vi "USBImageContinuousV1.3.vi"() -> ()   [LabVIEW 2017]
uses:
  C:/Program Files (x86)/National Instruments/LabVIEW 2019/ATMCD32D.dll
  <vilib>/Utility/file.llb/Write Delimited Spreadsheet (I64).vi
panel:
  in  "Tab Control":T1(tab)
  out "Expected position on spectrometer (pixels):":dbl
  in  "Harmonic":dbl min=10.0 max=40.0
  out "l (nm)":dbl
  out "E (J)":dbl
  out "E (eV)":dbl
  out "Nearest Harmonic of 800nm":dbl
  out "Cursor Position (pixels)":dbl
  out "Distance to nearest harmonic of 800nm (pixels)":dbl
  in  "Grating:":u16(ring) items=["Shimadzu 30-006  "]
  in  "Laser:":u16(ring) items=["800nm  "]
  in  "Trigger":u32(ring) items=["Internal", "External"]
  out "Initialize":u32
  in  "Exposure Time (secs)":sgl format="%.2f"
  out "Calculated Exposure Value":sgl format="%.5f"
  out "Get Acquired Data":u32
  out "Start Acquisition":u32
  out "Detector X Pixels":i32
  out "Check Timings":u32
  out "Set Acquisition Mode":u32
  out "Set Readout Mode":u32
  out "Set Trigger Mode":u32
  out "Set Exposure Time":u32
  out "Get Detector":u32
  out "Detector Y Pixels":i32
  out "Shut Down":u32
  out "Set Gate Mode":u32
  out "Set Image":u32
  out "Raw Image From Camera":i32[][](graph)
  out "Vertical Binned Waveform Graph":i32[](graph)
  out "Get Status":u32
  in  "Stop":bool
  in  "?":bool
  out "Camera Status:":bool
  out "Last Image Saved:":string
  in  "Caibration Date":u16(ring) items=["first calibration - 7/31", "7/31-current"]
  out "Caibration Date: indicator:":u16(ring) items=["first calibration - 7/31", "7/31-current"]
  out "Wavelength Graph (nm)":cluster{"No prefix":dbl, i32}[](graph)
  out "Energy Graph (eV)":cluster{"eV":dbl, i32}[](graph)
  out "Harmonics Graph":cluster{"No prefix":dbl, i32}[](graph)
  out "Status":u32
  # "Status"
  # "Return values"
  # "Acquisition Mode: Single Scan\nReadout Mode: Full Resolution Image"
  # "XUV Spectrometer Control VI"
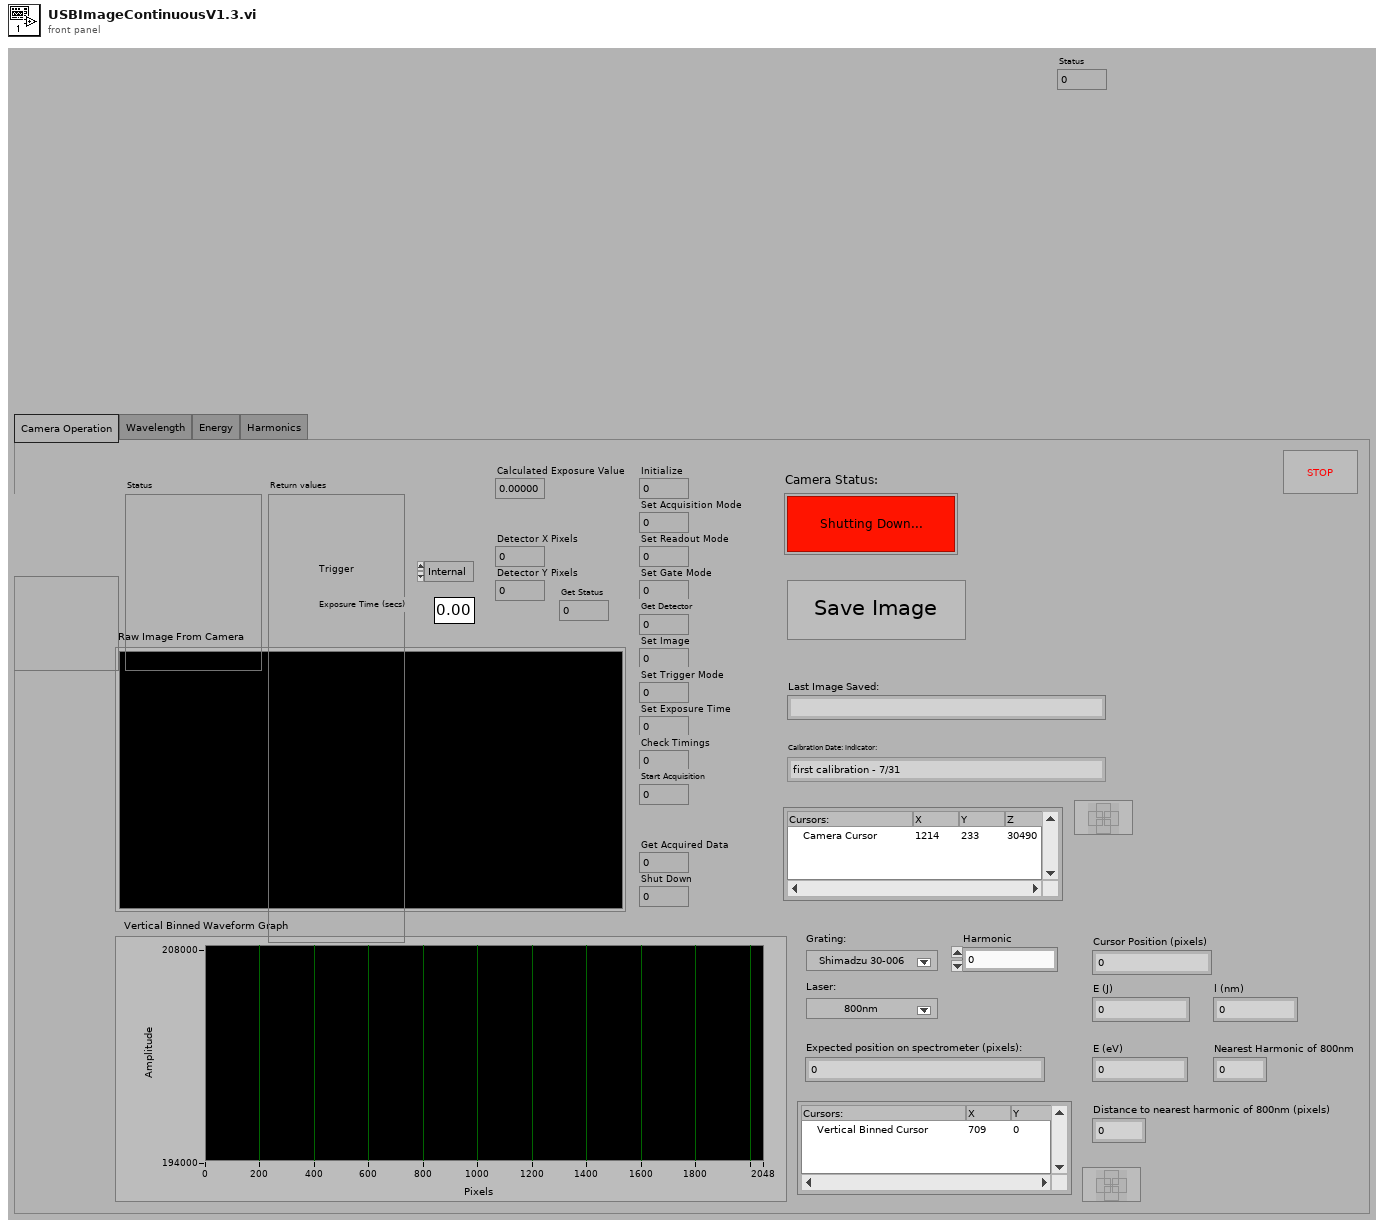
[diagram p1: front panel]
types:
  T1 = enum32{"Camera Operation", "Wavelength", "Energy", "Harmonics"}
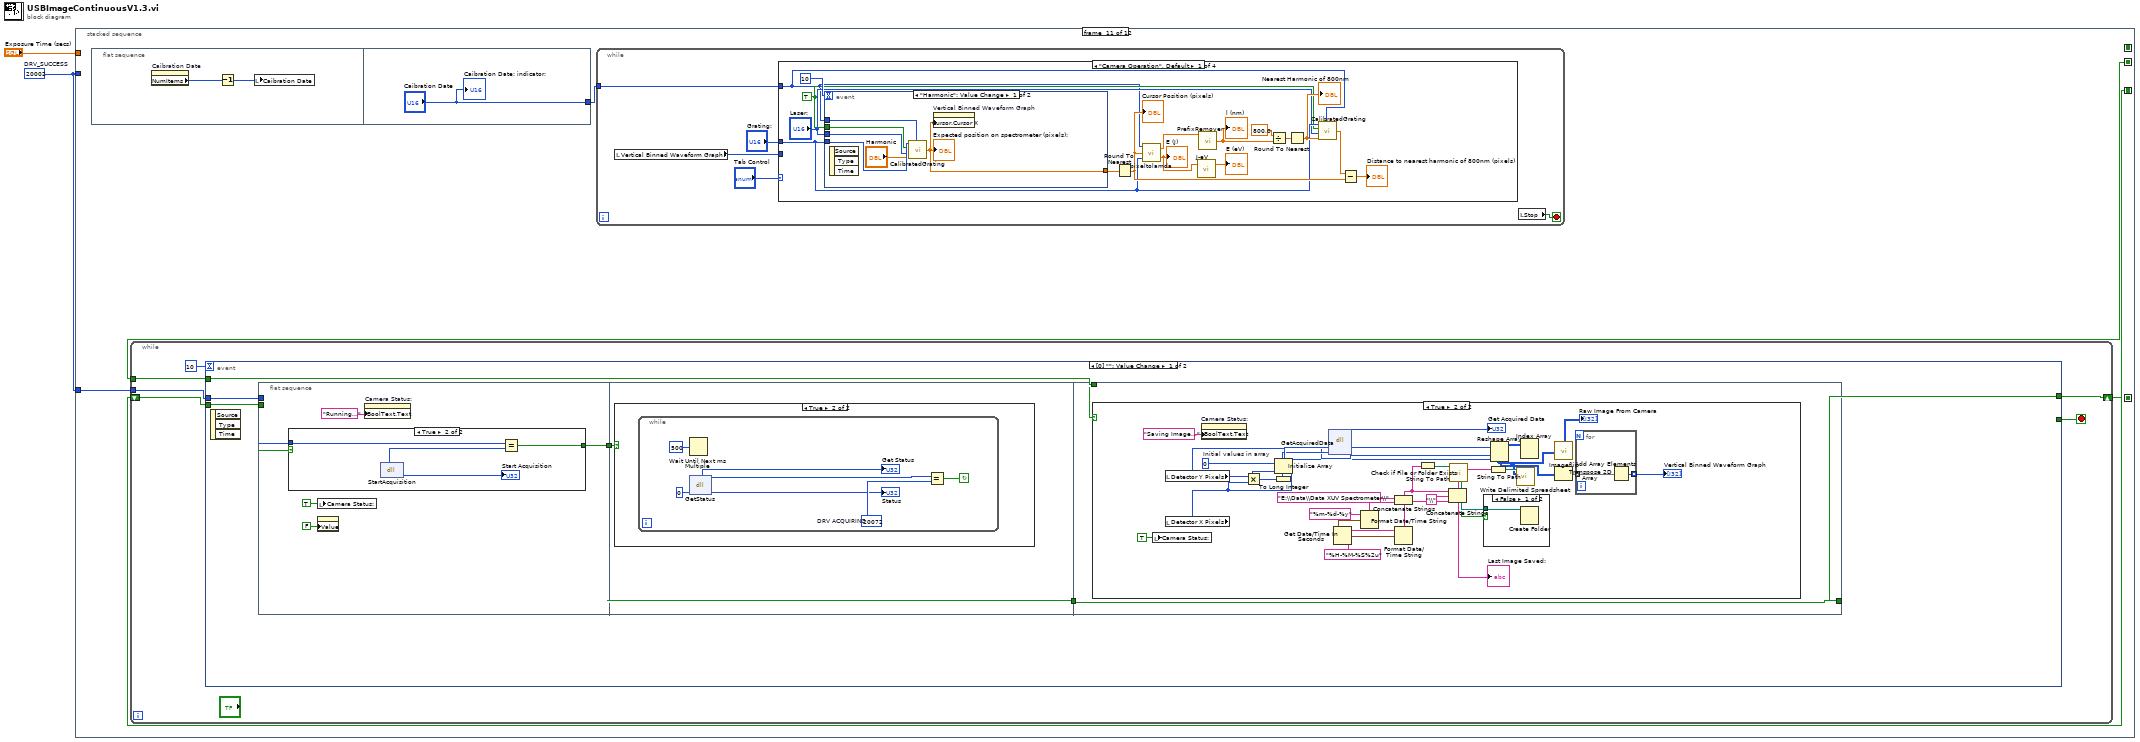
[diagram p0: block diagram]
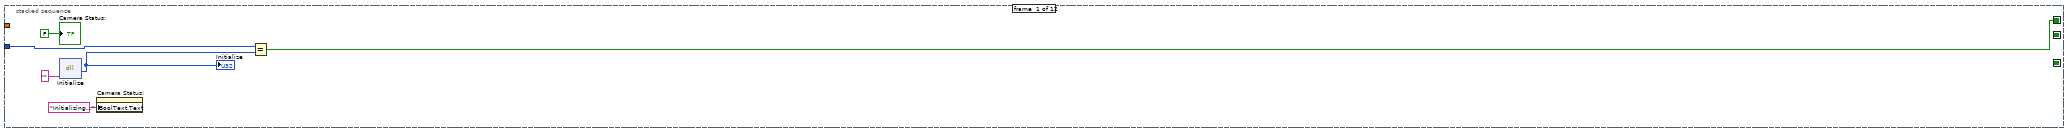
[diagram p2: hidden frame]
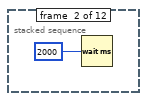
[diagram p3: hidden frame]
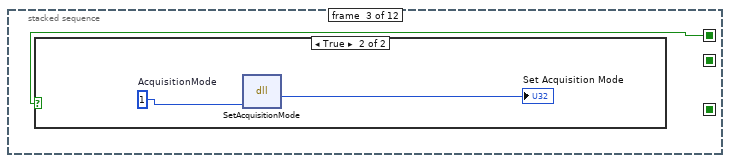
[diagram p4: hidden frame]
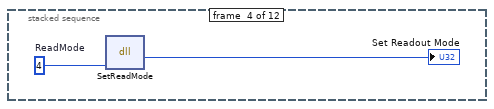
[diagram p6: hidden frame]
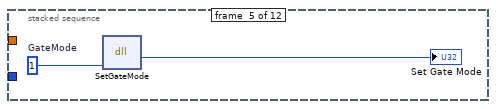
[diagram p7: hidden frame]
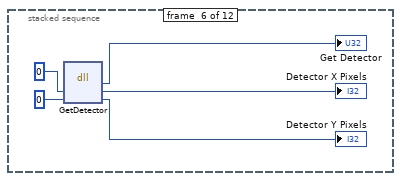
[diagram p8: hidden frame]
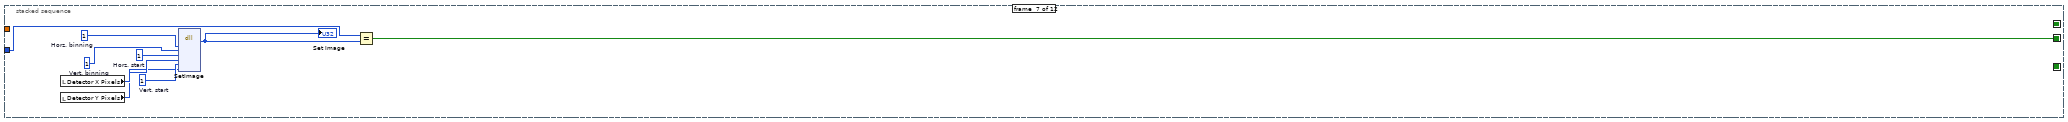
[diagram p9: hidden frame]
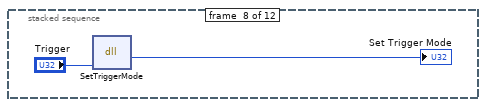
[diagram p10: hidden frame]
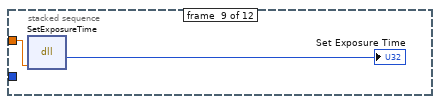
[diagram p11: hidden frame]
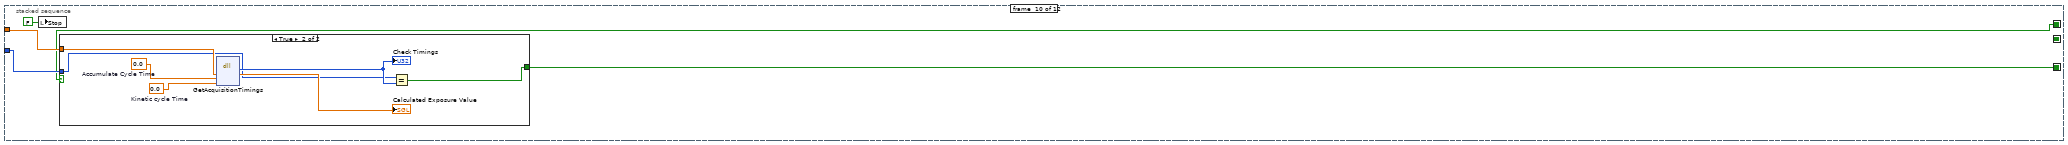
[diagram p12: hidden frame]
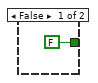
[diagram p13: hidden frame]
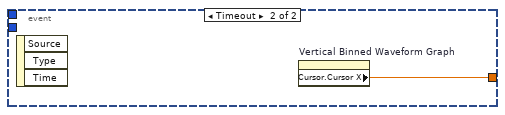
[diagram p14: hidden frame]
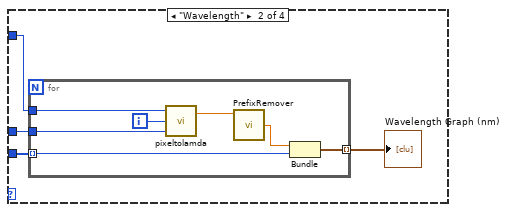
[diagram p15: hidden frame]
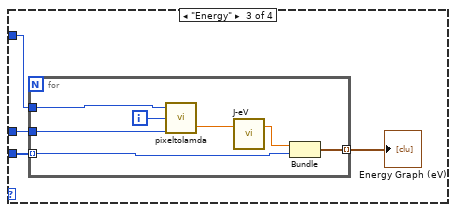
[diagram p16: hidden frame]
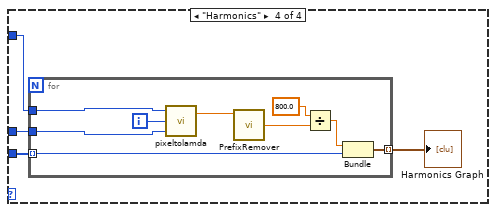
[diagram p17: hidden frame]
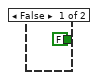
[diagram p18: hidden frame]
diagram:
  w1 = 20002  # DRV_SUCCESS
  n1 = stacked-sequence {
    seq-local: [w6 _ _ _ _ _ _ _ _ _ _ _] -> [_ _ w10 _ _ _ _ _ _ w36 _ w233]
    seq-local: [_ _ _ _ _ _ _ _ _ w37 _ _] -> [_ _ _ _ _ _ _ _ _ _ w52 _]
    seq-local: [_ _ _ _ _ _ _ _ _ _ w50 _] -> [_ _ _ _ _ _ _ _ _ _ _ _]
    seq-local: [_ _ _ _ _ _ w22 _ _ _ _ _] -> [_ _ _ _ _ _ _ _ _ _ w49 _]
    tunnel: "Exposure Time (secs)" -> [_ _ _ _ _ _ _ _ w34 w39 _ _]
    tunnel: w1 -> [w7 _ _ _ _ _ w24 _ _ w38 _ _]
    tunnel: w1 -> [_ _ _ _ _ _ _ _ _ _ w51 _]
    frame #0 {
      n2 = dll-call lib="C:/Program Files (x86)/National Instruments/LabVIEW 2019/atmcd32d.dll" fn="Initialize" label="Call Library Function Initialize"("") -> (w8:u32)  [unwired: 4 in, 2 out]
      "Initialize" <- w8
      n3 = property on="Camera Status:" class="Bool (strict)"("BoolText.Text"="Initializing..." ("String")) -> ()  [unwired: 2 in, 2 out]
      n4 = Equal?(x=w7, y=w8) -> (x = y?=w6:bool)
      "Camera Status:" <- FALSE ("Camera Status:")
    }
    frame #1 {
      n5 = Wait (ms)(milliseconds to wait=u32 2000) -> ()  [unwired: 1 out]
    }
    frame #2 {
      n6 = case shown="True" w10 {
        frame False {
        }
        frame True {
          w12 = u16 1  # AcquisitionMode
          n7 = dll-call lib="C:/Program Files (x86)/National Instruments/LabVIEW 2019/atmcd32d.dll" fn="SetAcquisitionMode" label="Call Library Function SetAcquisitionMode"(w12) -> (→"Set Acquisition Mode":u32)  [unwired: 4 in, 2 out]
        }
      }
    }
    frame #3 {
      w14 = u16 4  # ReadMode
      n8 = dll-call lib="C:/Program Files (x86)/National Instruments/LabVIEW 2019/atmcd32d.dll" fn="SetReadMode" label="Call Library Function SetReadMode"(w14) -> (→"Set Readout Mode":u32)  [unwired: 4 in, 2 out]
    }
    frame #4 {
      w16 = u16 1  # GateMode
      n9 = dll-call lib="C:/Program Files (x86)/National Instruments/LabVIEW 2019/atmcd32d.dll" fn="SetGateMode" label="Call Library Function SetGateMode"(w16) -> (→"Set Gate Mode":u32)  [unwired: 4 in, 2 out]
    }
    frame #5 {
      n10 = dll-call lib="C:/Program Files (x86)/National Instruments/LabVIEW 2019/atmcd32d.dll" fn="GetDetector" label="Call Library FunctionGetDetector"(i16 0, i16 0) -> (→"Get Detector":u32, →"Detector X Pixels":i32, →"Detector Y Pixels":i32)  [unwired: 3 in, 2 out]
    }
    frame #6 {
      w27 = u16 1  # Vert. start
      w28 = u16 1  # Horz. start
      w29 = u16 1  # Vert. binning
      w30 = u16 1  # Horz. binning
      n11 = local read "Detector X Pixels"() -> (w26:i32)
      n12 = local read "Detector Y Pixels"() -> (w25:i32)
      n13 = dll-call lib="C:/Program Files (x86)/National Instruments/LabVIEW 2019/atmcd32d.dll" fn="SetImage" label="Call Library Function SetImage"(w30, w29, w28, w26, w27, w25) -> (w23:u32)  [unwired: 9 in, 2 out]
      "Set Image" <- w23
      n14 = Equal?(x=w24, y=w23) -> (x = y?=w22:bool)
    }
    frame #7 {
      n15 = dll-call lib="C:/Program Files (x86)/National Instruments/LabVIEW 2019/atmcd32d.dll" fn="SetTriggerMode" label="Call Library Function SetTrigger Mode"("Trigger") -> (→"Set Trigger Mode":u32)  [unwired: 4 in, 2 out]
    }
    frame #8 {
      n16 = dll-call lib="C:/Program Files (x86)/National Instruments/LabVIEW 2019/atmcd32d.dll" fn="SetExposureTime" label="Call Library FunctionSet Exposure Time"(w34) -> (→"Set Exposure Time":u32)  [unwired: 4 in, 2 out]
    }
    frame #9 {
      n17 = local write "Stop"(FALSE ("Stop")) -> ()
      n18 = case shown="True" w36 {
        tunnel: w39 -> [_ w44]
        tunnel: w38 -> [_ w41]
        tunnel: [FALSE w43] -> w37
        frame False {
        }
        frame True {
          w46 = sgl 0.0  # Accumulate Cycle Time
          w47 = sgl 0.0  # Kinetic cycle Time
          n19 = dll-call lib="C:/Program Files (x86)/National Instruments/LabVIEW 2019/atmcd32d.dll" fn="GetAcquisitionTimings" label="Call Library Function Check Timings"(w44, w46, w47) -> (w42:u32, →"Calculated Exposure Value":sgl)  [unwired: 5 in, 2 out]
          "Check Timings" <- w42
          n20 = Equal?(x=w41, y=w42) -> (x = y?=w43:bool)
        }
      }
    }
    frame #10 {
      n21 = flat-sequence {
        tunnel: ["Caibration Date"] -> w48
        frame #0 {
          n22 = property on="Caibration Date" class="Ring (strict)"() -> ("NumItems"=w54:u32)  [unwired: 2 in, 2 out]
          n23 = Decrement(x=w54) -> (x-1=w53:u32)
          n24 = local write "Caibration Date"(w53) -> ()
        }
        frame #1 {
          "Caibration Date: indicator:" <- "Caibration Date"
        }
      }
      n25 = while {
        tunnel: w51 -> [w123]
        tunnel: w49 -> [w121]
        shift-right: [w122] -> w50
        shift-left: w52 -> [w124]
        stop <- w119 stop-if-true
        n26 = event shown="[0] \"\": Value Change" {
          selector: _ -> [_ _]
          dyn-events: _ -> [_ _]
          timeout: 10 -> [_ _]
          tunnel: w124 -> [w128 w185]
          tunnel: w123 -> [w127 w184]
          tunnel: [w126 w183] -> w122
          tunnel: w121 -> [w125 w182]
          tunnel: [_ w181] -> w119
          event Value Change {
            n27 = event-data() -> ()  [unwired: 1 in, 3 out]
            n28 = flat-sequence {
              tunnel: w128 -> [w136]
              tunnel: w127 -> [w135]
              tunnel: [w134] -> w130
              tunnel: w130 -> [w141]
              tunnel: [w141] -> w129
              tunnel: [w149] -> w126
              tunnel: w129 -> [w149]
              tunnel: w125 -> [w148]
              frame #0 {
                n29 = case shown="True" w136 {
                  tunnel: [FALSE w139] -> w134
                  tunnel: w135 -> [_ w138]
                  frame False {
                  }
                  frame True {
                    n30 = dll-call lib="C:/Program Files (x86)/National Instruments/LabVIEW 2019/atmcd32d.dll" fn="StartAcquisition" label="Call Library Function start acquisition"() -> (w140:u32)  [unwired: 3 in, 2 out]
                    "Start Acquisition" <- w140
                    n31 = Equal?(x=w138, y=w140) -> (x = y?=w139:bool)
                  }
                }
                n32 = local write "Camera Status:"(TRUE ("Camera Status:")) -> ()
                n33 = property class="Bool (strict)"("Value"=FALSE ("Take image")) -> ()  [unwired: 2 in, 2 out]
                n34 = property on="Camera Status:" class="Bool (strict)"("BoolText.Text"="Running..." ("Boolean Text.Text")) -> ()  [unwired: 2 in, 2 out]
              }
              frame #1 {
                n35 = case shown="True" w141 {
                  frame False {
                  }
                  frame True {
                    n36 = while {
                      stop <- w145 continue-if-true
                      w144 = u16 20072  # DRV ACQUIRING
                      n37 = Wait Until Next ms Multiple(millisecond multiple=u32 500) -> ()  [unwired: 1 out]
                      n38 = dll-call lib="C:/Program Files (x86)/National Instruments/LabVIEW 2019/atmcd32d.dll" fn="GetStatus" label="Call Library Function GetAcquisitionStatus"(u16 0) -> (→"Get Status":u32, w143:u32)  [unwired: 3 in, 2 out]
                      "Status" <- w143
                      n39 = Equal?(x=w143, y=w144) -> (x = y?=w145:bool)
                    }
                  }
                }
              }
              frame #2 {
                n40 = case shown="True" w148 {
                  frame False {
                  }
                  frame True {
                    w176 = 0  # Initial values in array
                    n41 = local write "Camera Status:"(TRUE ("Camera Status:")) -> ()
                    n42 = local read "Detector Y Pixels"() -> (w170:i32)
                    n43 = local read "Detector X Pixels"() -> (w169:i32)
                    n44 = property on="Camera Status:" class="Bool (strict)"("BoolText.Text"="Saving Image..." ("Boolean Text.Text")) -> ()  [unwired: 2 in, 2 out]
                    n45 = Multiply(x=w170, y=w169) -> (x*y=w172:i32)
                    n46 = To Long Integer(number=w172) -> (32bit integer=w173:i32)
                    n47 = Initialize Array "Initialize Array"(w176, w172) -> (w174:i32[])
                    n48 = dll-call lib="C:/Program Files (x86)/National Instruments/LabVIEW 2019/atmcd32d.dll" fn="GetAcquiredData" label="Call Library Function Get Acquired data"(w174, w173) -> (→"Get Acquired Data":u32, w171:i32[])  [unwired: 4 in, 2 out]
                    n49 = Get Date/Time In Seconds() -> (seconds since 1Jan1904=w166:timestamp)
                    n50 = Format Date/Time String(time format string (%c)="%m-%d-%y", seconds (now)=w166) -> (date/time string=w164:string)  [unwired: 1 in]
                    n51 = Concatenate Strings("E:\\Data\\Data XUV Spectrometer\\" ("string"), w164) -> (w167:string)
                    n52 = Format Date/Time String(time format string (%c)="%H-%M-%S%2u", seconds (now)=w166) -> (date/time string=w165:string)  [unwired: 1 in]
                    n53 = String To Path(string=w167) -> (path=w163:path)
                    n54 = Concatenate Strings(w167, "\\" ("string"), w165) -> (w168:string)
                    "Last Image Saved:" <- w168
                    n55 = call <vilib>:"Check if File or Folder Exists.vi"("path"=w163) -> ("file or folder exists?"=w161:bool, "dup path"=w162:path)  [unwired: 8 in, 1 out]
                    n56 = case shown="False" w161 {
                      tunnel: w162 -> [w179 _]
                      frame False {
                        n57 = Create Folder(path (use dialog)=w179) -> ()  [unwired: 2 in, 3 out]
                      }
                      frame True {
                      }
                    }
                    n58 = String To Path(string=w168) -> (path=w156:path)
                    n59 = Reshape Array(w171, w170, w169) -> (w151:i32[][])
                    n60 = call-poly <vilib>:"Write Delimited Spreadsheet.vi"("file path (dialog if empty)"=w156, "2D data"=w151) -> ()  [unwired: 12 in, 2 out]
                    n61 = Index Array(array=w151) -> ()  [unwired: 2 in, 1 out]
                    n62 = call "Imageflip.vi"("2D array"=w151) -> ("transposed array"=→"Raw Image From Camera":i32[][])
                    n63 = Transpose 2D Array(2D array=w151) -> (transposed array=w155:i32[][])
                    n64 = for {
                      tunnel: w155 -> [w178] mode=indexing
                      tunnel: [w177] -> w154 mode=indexing
                      n65 = Add Array Elements(numeric array=w178) -> (sum=w177:i32)
                    }
                    "Vertical Binned Waveform Graph" <- w154
                  }
                }
              }
            }
          }
          event Timeout {
            n66 = event-data() -> ()  [unwired: 1 in, 3 out]
            n67 = flat-sequence {
              tunnel: w185 -> [w192]
              tunnel: w184 -> [w191]
              tunnel: [w190] -> w187
              tunnel: w187 -> [w197]
              tunnel: [w197] -> w186
              tunnel: w186 -> [w204]
              tunnel: w182 -> [w205]
              tunnel: [w204] -> w180
              tunnel: ["Stop"] -> w181
              tunnel: [w230] -> w183
              tunnel: w180 -> [w230]
              frame #0 {
                n68 = case shown="True" w192 {
                  tunnel: [FALSE w196] -> w190
                  tunnel: w191 -> [_ w195]
                  frame False {
                  }
                  frame True {
                    n69 = dll-call lib="C:/Program Files (x86)/National Instruments/LabVIEW 2019/atmcd32d.dll" fn="StartAcquisition" label="Call Library Function start acquisition"() -> (w194:u32)  [unwired: 3 in, 2 out]
                    n70 = local write "Start Acquisition"(w194) -> ()
                    n71 = Equal?(x=w195, y=w194) -> (x = y?=w196:bool)
                  }
                }
                n72 = local write "Camera Status:"(TRUE ("Camera Status:")) -> ()
                n73 = property on="Camera Status:" class="Bool (strict)"("BoolText.Text"="Running..." ("Boolean Text.Text")) -> ()  [unwired: 2 in, 2 out]
              }
              frame #1 {
                n74 = case shown="True" w197 {
                  frame False {
                  }
                  frame True {
                    n75 = while {
                      stop <- w201 continue-if-true
                      w200 = u16 20072  # DRV ACQUIRING
                      n76 = Wait Until Next ms Multiple(millisecond multiple=u32 500) -> ()  [unwired: 1 out]
                      n77 = dll-call lib="C:/Program Files (x86)/National Instruments/LabVIEW 2019/atmcd32d.dll" fn="GetStatus" label="Call Library Function GetAcquisitionStatus"(u16 0) -> (w199:u32, w198:u32)  [unwired: 3 in, 2 out]
                      n78 = local write "Status"(w198) -> ()
                      n79 = local write "Get Status"(w199) -> ()
                      n80 = Equal?(x=w198, y=w200) -> (x = y?=w201:bool)
                    }
                  }
                }
              }
              frame #2 {
                n81 = case shown="True" w205 {
                  frame False {
                  }
                  frame True {
                    w220 = 0  # Initial values in array
                    n82 = local read "Detector Y Pixels"() -> (w215:i32)
                    n83 = local read "Detector X Pixels"() -> (w214:i32)
                    n84 = Multiply(x=w215, y=w214) -> (x*y=w217:i32)
                    n85 = Initialize Array "Initialize Array"(w220, w217) -> (w219:i32[])
                    n86 = To Long Integer(number=w217) -> (32bit integer=w218:i32)
                    n87 = dll-call lib="C:/Program Files (x86)/National Instruments/LabVIEW 2019/atmcd32d.dll" fn="GetAcquiredData" label="Call Library Function Get Acquired data"(w219, w218) -> (w212:u32, w216:i32[])  [unwired: 4 in, 2 out]
                    n88 = local write "Get Acquired Data"(w212) -> ()
                    n89 = Reshape Array(w216, w215, w214) -> (w206:i32[][])
                    n90 = Index Array(array=w206) -> ()  [unwired: 2 in, 1 out]
                    n91 = Array Max & Min(array=w206) -> (max value=w210:i32)  [unwired: 3 out]
                    n92 = Transpose 2D Array(2D array=w206) -> (transposed array=w213:i32[][])
                    n93 = call "Imageflip.vi"("2D array"=w206) -> ("transposed array"=w207:i32[][])
                    n94 = for {
                      tunnel: w213 -> [w228] mode=indexing
                      tunnel: [w227] -> w211 mode=indexing
                      n95 = Add Array Elements(numeric array=w228) -> (sum=w227:i32)
                    }
                    n96 = local write "Raw Image From Camera"(w207) -> ()
                    n97 = Greater?(x=w210, y=64900) -> (0:w208:bool)
                    n98 = case shown="True" w208 {
                      frame False {
                      }
                      frame True {
                        n99 = local write "Camera Status:"(FALSE ("Camera Status:")) -> ()
                        n100 = property on="Camera Status:" class="Bool (strict)"("BoolText.Text"="Saturated!" ("Boolean Text.Text")) -> ()  [unwired: 2 in, 2 out]
                        n101 = Two Button Dialog(message="Camera is saturating! Reduce photon flux!", 1:"I've fixed it, and I want to continue" ("message"), 2:"Shut Down Camera" ("T button name (\"OK\")")) -> (T button?=w222:bool)
                        n102 = local write "Stop"(w222) -> ()
                      }
                    }
                    n103 = local write "Vertical Binned Waveform Graph"(w211) -> ()
                  }
                }
              }
              frame #3 {
              }
            }
          }
        }
      }
      n104 = while {
        tunnel: w48 -> [w56]
        stop <- w57 stop-if-true
        n105 = local read "Vertical Binned Waveform Graph"() -> (w59:i32[])
        n106 = case shown="\"Camera Operation\", Default" "Tab Control" {
          tunnel: w59 -> [_ w87 w98 w109]
          tunnel: "Grating:" -> [w64 w86 w97 w108]
          tunnel: w56 -> [w61 w84 w95 w106]
          frame "Camera Operation", Default {
            w63 = TRUE
            n107 = event shown="[0] \"Harmonic\": Value Change" {
              selector: _ -> [_ _]
              dyn-events: _ -> [_ _]
              timeout: 10 -> [_ _]
              tunnel: [w78 w83] -> w65
              tunnel: w64 -> [w82 _]
              tunnel: w63 -> [w81 _]
              tunnel: "Laser:" -> [w80 _]
              tunnel: w61 -> [w79 _]
              event "Harmonic": Value Change {
                n108 = event-data() -> ()  [unwired: 1 in, 3 out]
                n109 = call "CalibratedGrating.vi"("Grating:"=w82, "Subvi?"=w81, "Laser:"=w80, "Harmonic"="Harmonic", "Caibration Date"=w79) -> ("Position on spectrometer (pixels):"=w78:dbl)
                "Expected position on spectrometer (pixels):" <- w78
                n110 = property on="Vertical Binned Waveform Graph" class="WFGraph (strict)"("Cursor.Cursor X"=w78) -> ()  [unwired: 2 in, 2 out]
              }
              event Timeout {
                n111 = event-data() -> ()  [unwired: 1 in, 3 out]
                n112 = property on="Vertical Binned Waveform Graph" class="WFGraph (strict)"() -> ("Cursor.Cursor X"=w83:dbl)  [unwired: 2 in, 2 out]
              }
            }
            n113 = Round To Nearest(number=w65) -> (nearest integer value=w70:dbl)
            "Cursor Position (pixels)" <- w70
            n114 = call "pixeltolamda.vi"("Grating:"=w64, "Pixel Postion"=w70, "Caibration Date"=w61) -> ("E (J)"=w72:dbl, "lamda (m)"=w76:dbl)
            "E (J)" <- w72
            n115 = call "J-eV.vi"("J"=w72) -> ("eV"=→"E (eV)":dbl)  [unwired: 1 in, 1 out]
            n116 = call "PrefixRemover.vi"("Nano"=w76) -> ("No prefix"=w73:dbl)  [unwired: 3 in]
            "l (nm)" <- w73
            n117 = Divide(x=800.0, y=w73) -> (x/y=w75:dbl)
            n118 = Round To Nearest(number=w75) -> (nearest integer value=w69:dbl)
            "Nearest Harmonic of 800nm" <- w69
            n119 = call "CalibratedGrating.vi"("Grating:"=w64, "Subvi?"=w63, "Laser:"="Laser:", "Harmonic"=w69, "Caibration Date"=w61) -> ("Position on spectrometer (pixels):"=w68:dbl)
            n120 = Subtract(x=w68, y=w70) -> (x-y=→"Distance to nearest harmonic of 800nm (pixels)":dbl)
          }
          frame "Wavelength" {
            n121 = for {
              tunnel: w87 -> [w90] mode=indexing
              tunnel: w86 -> [w92]
              tunnel: [w89] -> w85 mode=indexing
              tunnel: w84 -> [w88]
              i -> [w91]
              n122 = call "pixeltolamda.vi"("Grating:"=w92, "Pixel Postion"=w91, "Caibration Date"=w88) -> ("lamda (m)"=w93:dbl)  [unwired: 1 out]
              n123 = call "PrefixRemover.vi"("Nano"=w93) -> ("No prefix"=w94:dbl)  [unwired: 3 in]
              n124 = Bundle("No prefix"=w94, w90) -> (w89:cluster{"No prefix":dbl, i32})  [unwired: 1 in]
            }
            "Wavelength Graph (nm)" <- w85
          }
          frame "Energy" {
            n125 = for {
              tunnel: w98 -> [w101] mode=indexing
              tunnel: w97 -> [w104]
              tunnel: [w100] -> w96 mode=indexing
              tunnel: w95 -> [w99]
              i -> [w105]
              n126 = call "pixeltolamda.vi"("Grating:"=w104, "Pixel Postion"=w105, "Caibration Date"=w99) -> ("E (J)"=w103:dbl)  [unwired: 1 out]
              n127 = call "J-eV.vi"("J"=w103) -> ("eV"=w102:dbl)  [unwired: 1 in, 1 out]
              n128 = Bundle("eV"=w102, w101) -> (w100:cluster{"eV":dbl, i32})  [unwired: 1 in]
            }
            "Energy Graph (eV)" <- w96
          }
          frame "Harmonics" {
            n129 = for {
              tunnel: w109 -> [w115] mode=indexing
              tunnel: w108 -> [w117]
              tunnel: [w114] -> w107 mode=indexing
              tunnel: w106 -> [w110]
              i -> [w116]
              n130 = call "pixeltolamda.vi"("Grating:"=w117, "Pixel Postion"=w116, "Caibration Date"=w110) -> ("lamda (m)"=w118:dbl)  [unwired: 1 out]
              n131 = call "PrefixRemover.vi"("Nano"=w118) -> ("No prefix"=w112:dbl)  [unwired: 3 in]
              n132 = Divide(x=800.0, y=w112) -> (x/y=w111:dbl)
              n133 = Bundle(w111, w115) -> (w114:cluster{dbl, i32})  [unwired: 1 in]
            }
            "Harmonics Graph" <- w107
          }
        }
        n134 = local read "Stop"() -> (w57:bool)
      }
    }
    frame #11 {
      n135 = local write "Camera Status:"(FALSE ("Camera Status:")) -> ()
      n136 = property on="Camera Status:" class="Bool (strict)"("BoolText.Text"="Shutting Down..." ("Boolean Text.Text")) -> ()  [unwired: 2 in, 2 out]
      n137 = case shown="True" w233 {
        frame False {
        }
        frame True {
          n138 = dll-call lib="C:/Program Files (x86)/National Instruments/LabVIEW 2019/atmcd32d.dll" fn="ShutDown" label="Call Library Function Shutdown"() -> (→"Shut Down":u32)  [unwired: 3 in, 2 out]
        }
      }
    }
  }
